vi "kalmanR_v.vi"(5 "error in (no error)":errorcluster) -> (16 "R_v":T1, 19 "error out":errorcluster)   [LabVIEW 2023, in "Vision.lvclass"]
uses:
  Vision.lvclass
  <vilib>/Analysis/Matrix/Datatypes/RealMatrix.ctl
  <vilib>/Analysis/Matrix/NI_Matrix.lvlib
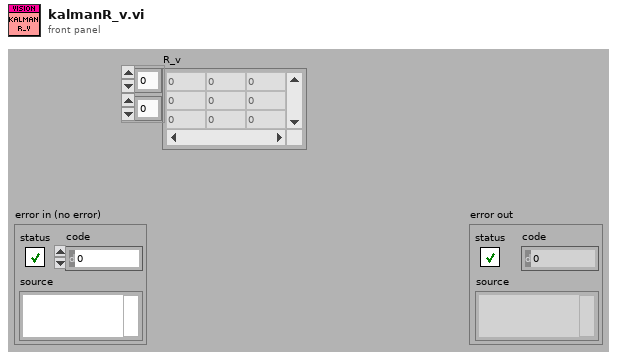
[diagram p1: front panel]
types:
  T1 = typedef "NI_Matrix.lvlib/RealMatrix.ctl" = dbl[][]
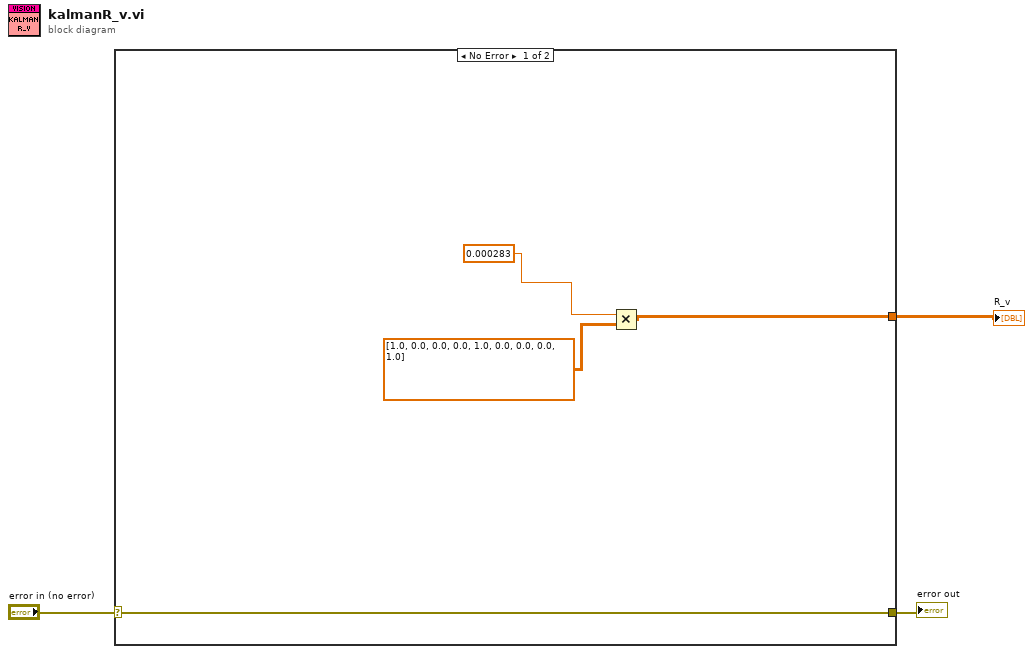
[diagram p0: block diagram]
diagram:
  n1 = case shown="No Error" "error in (no error)" {
    selector: "error in (no error)" -> [w7 w8]
    tunnel: [w7 w8] -> w2
    tunnel: [w4 _] -> w1
    frame No Error {
      n2 = Multiply(x=0.000283, y=dbl[][] [[1.0, 0.0, 0.0], [0.0, 1.0, 0.0], [0.0, 0.0, 1.0]]) -> (x*y=w4:dbl[][])
    }
    frame Error {
    }
  }
  "error out" <- w2
  "R_v" <- w1
